vi "T564_TriggerImpedanceFromSETresponse.vi"(11 "String":string) -> (3 "Impedance":T1)   [LabVIEW 2013]
uses:
  TypeDefs/TriggerImpedance.ctl
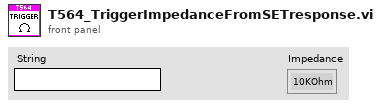
[diagram p1: front panel]
types:
  T1 = typedef "TriggerImpedance.ctl" = enum16{"10KOhm", "50Ohms"}
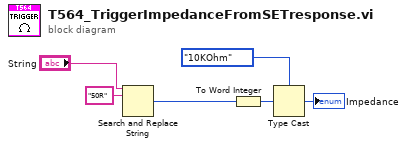
[diagram p0: block diagram]
diagram:
  n1 = Search and Replace String(input string="String", search string="50R") -> (number of replacements=w3:i32)  [unwired: 6 in, 3 out]
  n2 = To Word Integer(number=w3) -> (16bit integer=w6:i16)
  n3 = Type Cast(type=TriggerImpedance."10KOhm" ("Impedance"), x=w6) -> (*(type *) &x=→"Impedance":T1)
